vi "dfd_Render Real Root+.vi"(0 "Negative Exponent?":bool=TRUE, 4 "alignment(left, top)":T1, 5 "format string":string="%#g", 6 "bracket":cluster{"left":string, "right":string}={"left"="(", "right"=")"}, 7 "Fonts Input":T2(array[cluster]), 8 "variable":string="z", 9 "origin":cluster{"x":i16, "y":i16}, 10 "coefficients":dbl[](array[numeric]) format="%.2f", 11 "new picture":picture) -> (2 "text rect":T3, 3 "picture out":picture)   [LabVIEW 2017, in "NI_DigFilter_Process.lvlib"]
uses:
  <vilib>/addons/Digital Filter Design/NI_DigFilter_Process.lvlib
  <vilib>/Analysis/polynomials.llb/Unique Numbers and Multiplicity (DBL).vi
  <vilib>/Analysis/NI_AALPro.lvlib
panel:
  in  "Fonts Defaut":T2(array[cluster])=[{"Font Name:"="Tahoma", "Size"=13, "Strikeout?"=FALSE, "Italic?"=FALSE, "Underline?"=FALSE, "Outline?"=FALSE, "Shadow?"=FALSE, "Bold?"=FALSE}, {"Font Name:"="Tahoma", "Size"=13, "Strikeout?"=FALSE, "Italic?"=FALSE, "Underline?"=FALSE, "Outline?"=FALSE, "Shadow?"=FALSE, "Bold?"=FALSE}, {"Font Name:"="Tahoma", "Size"=11, "Strikeout?"=FALSE, "Italic?"=FALSE, "Underline?"=FALSE, "Outline?"=FALSE, "Shadow?"=FALSE, "Bold?"=FALSE}]
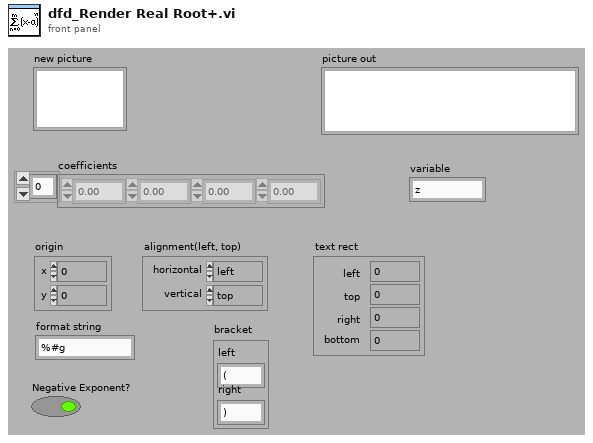
[diagram p1: front panel]
types:
  T1 = cluster{"horizontal":enum16{"left", "center", "right"}, "vertical":enum16{"top", "center", "bottom"}}
  T2 = cluster{"Font Name:":string, "Size":i16, "Strikeout?":bool, "Italic?":bool, "Underline?":bool, "Outline?":bool, "Shadow?":bool, "Bold?":bool}[]
  T3 = cluster{"left":i16, "top":i16, "right":i16, "bottom":i16}
  T4 = enum16{"User-specified Font", "Application Font", "System Font", "Dialog Font"}
  T5 = cluster{"Font Name:":string, "Size":i16, "Strikeout?":bool, "Italic?":bool, "Underline?":bool, "Outline?":bool, "Shadow?":bool, "Bold?":bool}
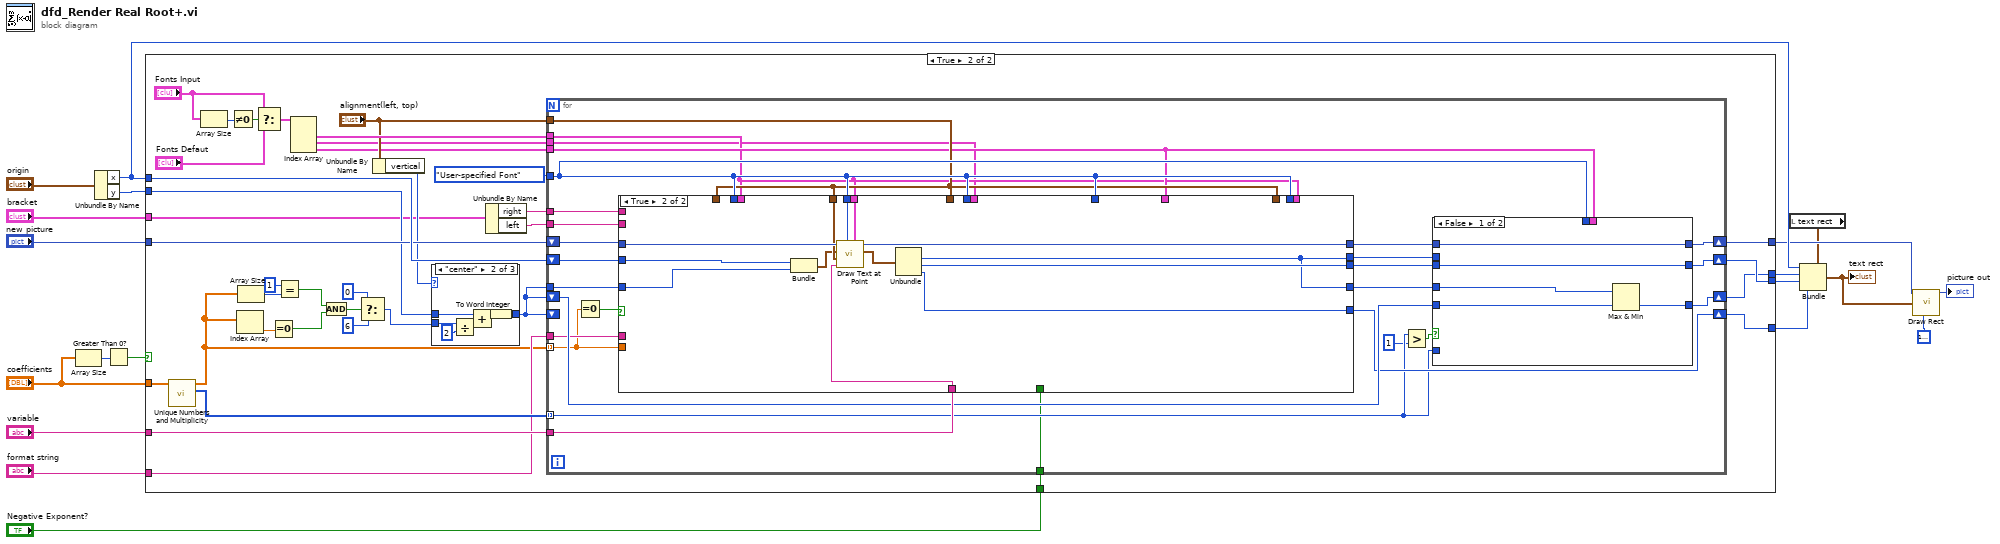
[diagram p0: block diagram]
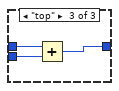
[diagram p4: hidden frame]
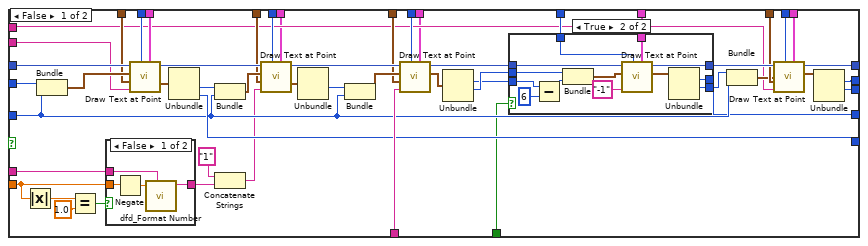
[diagram p5: hidden frame]
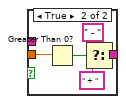
[diagram p7: hidden frame]
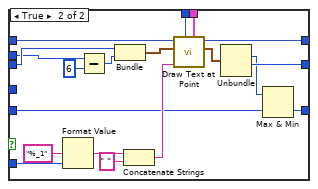
[diagram p8: hidden frame]
diagram:
  n1 = Array Size(array="coefficients") -> (size(s)=w12:i32)
  n2 = Unbundle By Name("origin") -> ("x"=w17:i16, "y"=w15:i16)
  n3 = Greater Than 0?(x=w12) -> (x > 0?=w11:bool)
  n4 = case shown="True" w11 {
    tunnel: [w22 w59] -> w19
    tunnel: [w21 w58] -> w18
    tunnel: w17 -> [w22 w56]
    tunnel: [w21 w55] -> w16
    tunnel: w15 -> [w21 w43]
    tunnel: [w20 w49] -> w7
    tunnel: "coefficients" -> [_ w47]
    tunnel: "new picture" -> [w20 w46]
    tunnel: "Negative Exponent?" -> [_ w38]
    tunnel: "variable" -> [_ w37]
    tunnel: "format string" -> [_ w36]
    tunnel: "bracket" -> [_ w35]
    frame False {
    }
    frame True {
      n5 = call-poly <vilib>:"Unique Numbers and Multiplicity.vi"("Numbers"=w47) -> ("Multiplicity"=w45:u32[], "Unique Numbers"=w32:dbl[])  [unwired: 9 out]
      n6 = Array Size(array="Fonts Input") -> (size(s)=w53:i32)
      n7 = Not Equal To 0?(x=w53) -> (x != 0?=w54:bool)
      n8 = Index Array(array=w32) -> (element=w31:dbl)  [unwired: 1 in]
      n9 = Array Size(array=w32) -> (size(s)=w30:i32)
      n10 = Select(t="Fonts Input", s=w54, f="Fonts Defaut") -> (s? t:f=w51:T2)
      n11 = Equal To 0?(x=w31) -> (x = 0?=w27:bool)
      n12 = Equal?(x=1, y=w30) -> (x = y?=w28:bool)
      n13 = Index Array(array=w51) -> (element #1=w48:T5, element #2=w40:T5, element #3=w39:T5)  [unwired: 3 in]
      n14 = And(x=w28, y=w27) -> (x .and. y?=w26:bool)
      n15 = Select(t=i16 0, s=w26, f=i16 6) -> (s? t:f=w24:i16)
      n16 = Unbundle By Name("alignment(left, top)") -> ("vertical"=w41:enum16{"top", "center", "bottom"})
      n17 = case shown="\"center\"" w41 {
        tunnel: [w60 w61 w68] -> w42
        tunnel: w43 -> [w60 w66 w69]
        tunnel: w24 -> [_ w64 w67]
        frame "bottom", Default {
        }
        frame "center" {
          n18 = Divide(x=w64, y=i16 2) -> (x/y=w62:dbl)
          n19 = Add(x=w66, y=w62) -> (x+y=w65:dbl)
          n20 = To Word Integer(number=w65) -> (16bit integer=w61:i16)
        }
        frame "top" {
          n21 = Add(x=w69, y=w67) -> (x+y=w68:i16)
        }
      }
      n22 = Unbundle By Name(w35) -> ("right"=w33:string, "left"=w34:string)
      n23 = for {
        tunnel: w32 -> [w81] mode=indexing
        shift-right: [w90] -> w49
        shift-left: w46 -> [w95]
        tunnel: w37 -> [w96]
        shift-right: [w89] -> w59
        shift-left: w56 -> [w94]
        tunnel: w42 -> [w92]
        shift-right: [w88] -> w58
        shift-left: w42 -> [w93]
        tunnel: T4."User-specified Font" ("desired font(Application)") -> [w80]
        shift-right: [w87] -> w55
        shift-left: w42 -> [_]
        tunnel: w36 -> [w91]
        tunnel: "alignment(left, top)" -> [w79]
        tunnel: w48 -> [w71]
        tunnel: w45 -> [w86] mode=indexing
        tunnel: w40 -> [w70]
        tunnel: w39 -> [w76]
        tunnel: w38 -> [w77]
        tunnel: w34 -> [w74]
        tunnel: w33 -> [w73]
        n24 = Equal To 0?(x=w81) -> (x = 0?=w78:bool)
        n25 = case shown="True" w78 {
          tunnel: w96 -> [w127 w185]
          tunnel: w79 -> [w128 _]
          tunnel: w95 -> [w147 w184]
          tunnel: w94 -> [w146 w180]
          tunnel: w92 -> [w111 w177]
          tunnel: w91 -> [w145 _]
          tunnel: [w123 w176] -> w87
          tunnel: [w117 w181] -> w85
          tunnel: [w115 w175] -> w84
          tunnel: w80 -> [w134 _]
          tunnel: w81 -> [w126 _]
          tunnel: w71 -> [w135 _]
          tunnel: w80 -> [w120 _]
          tunnel: w80 -> [w133 w182]
          tunnel: w80 -> [w132 _]
          tunnel: w79 -> [w131 _]
          tunnel: w79 -> [w129 w183]
          tunnel: w71 -> [w114 _]
          tunnel: w80 -> [w113 _]
          tunnel: w79 -> [w112 _]
          tunnel: w76 -> [w109 _]
          tunnel: w77 -> [w108 _]
          tunnel: [w106 w174] -> w75
          tunnel: w74 -> [w99 _]
          tunnel: w73 -> [w101 _]
          tunnel: [w100 w174] -> w72
          tunnel: w71 -> [w98 w173]
          tunnel: w70 -> [w97 _]
          frame False {
            n26 = Absolute Value(x=w126) -> (abs(x)=w107:dbl)
            n27 = Bundle("x"=w146, "y"=w111) -> (w138:cluster{"x":i16, "y":i16})  [unwired: 1 out]
            n28 = Equal?(x=w107, y=1.0) -> (x = y?=w124:bool)
            n29 = case shown="False" w124 {
              tunnel: w145 -> [w167 _]
              tunnel: [w166 w169] -> w104
              tunnel: w126 -> [w165 w170]
              frame False {
                n30 = Negate(x=w165) -> (-x=w164:dbl)
                n31 = call <vilib>:"dfd_Format Number.vi"("format string"=w167, "Coefficient"=w164) -> ("String Coefficient"=w166:string)  [unwired: 9 out]
              }
              frame True {
                n32 = Greater Than 0?(x=w170) -> (x > 0?=w171:bool)
                n33 = Select(t=" - " ("string"), s=w171, f=" + ") -> (s? t:f=w169:string)
              }
            }
            n34 = call <vilib>:"Draw Text at Point.vi"("[user-specified font]"=w135, "desired font(Application)"=w132, "text"=w99, "alignment(left, top)"=w131, "origin"=w138, "picture"=w147) -> ("text rect"=w142:T3, "new picture"=w143:picture)  [unwired: 3 in, 1 out]
            n35 = Unbundle(w142) -> ("right"=w140:i16, "bottom"=w123:i16)  [unwired: 2 out]
            n36 = Bundle("right"=w140, "y"=w111) -> (w130:cluster{"right":i16, "y":i16})  [unwired: 1 out]
            n37 = Concatenate Strings("1" ("string"), w104) -> (w102:string)
            n38 = call <vilib>:"Draw Text at Point.vi"("[user-specified font]"=w98, "desired font(Application)"=w133, "text"=w102, "alignment(left, top)"=w129, "origin"=w130, "picture"=w143) -> ("text rect"=w141:T3, "new picture"=w136:picture)  [unwired: 3 in, 1 out]
            n39 = Unbundle(w141) -> ("right"=w139:i16)  [unwired: 3 out]
            n40 = Bundle("right"=w139, "y"=w111) -> (w137:cluster{"right":i16, "y":i16})  [unwired: 1 out]
            n41 = call <vilib>:"Draw Text at Point.vi"("[user-specified font]"=w97, "desired font(Application)"=w134, "text"=w127, "alignment(left, top)"=w128, "origin"=w137, "picture"=w136) -> ("text rect"=w144:T3, "new picture"=w122:picture)  [unwired: 3 in, 1 out]
            n42 = Unbundle(w144) -> ("top"=w105:i16, "right"=w121:i16)  [unwired: 2 out]
            n43 = case shown="True" w108 {
              tunnel: w122 -> [w150 w159]
              tunnel: w121 -> [w149 w158]
              tunnel: w109 -> [_ w157]
              tunnel: [w150 w155] -> w118
              tunnel: [w149 w154] -> w116
              tunnel: w120 -> [_ w153]
              tunnel: [w148 w152] -> w106
              tunnel: w105 -> [w148 w151]
              frame False {
              }
              frame True {
                n44 = Subtract(x=w151, y=i16 6) -> (x-y=w162:i16)
                n45 = Bundle("right"=w158, w162) -> (w163:cluster{"right":i16, i16})  [unwired: 1 out]
                n46 = call <vilib>:"Draw Text at Point.vi"("[user-specified font]"=w157, "desired font(Application)"=w153, "text"="-1", "origin"=w163, "picture"=w159) -> ("text rect"=w160:T3, "new picture"=w155:picture)  [unwired: 4 in, 1 out]
                n47 = Unbundle(w160) -> ("top"=w152:i16, "right"=w154:i16)  [unwired: 2 out]
              }
            }
            n48 = Bundle("right"=w116, "y"=w111) -> (w110:cluster{"right":i16, "y":i16})  [unwired: 1 out]
            n49 = call <vilib>:"Draw Text at Point.vi"("[user-specified font]"=w114, "desired font(Application)"=w113, "text"=w101, "alignment(left, top)"=w112, "origin"=w110, "picture"=w118) -> ("text rect"=w119:T3, "new picture"=w117:picture)  [unwired: 3 in, 1 out]
            n50 = Unbundle(w119) -> ("top"=w100:i16, "right"=w115:i16)  [unwired: 2 out]
          }
          frame True {
            n51 = Bundle("x"=w180, "y"=w177) -> (w179:cluster{"x":i16, "y":i16})  [unwired: 1 out]
            n52 = call <vilib>:"Draw Text at Point.vi"("[user-specified font]"=w173, "desired font(Application)"=w182, "text"=w185, "alignment(left, top)"=w183, "origin"=w179, "picture"=w184) -> ("text rect"=w178:T3, "new picture"=w181:picture)  [unwired: 3 in, 1 out]
            n53 = Unbundle(w178) -> ("top"=w174:i16, "right"=w175:i16, "bottom"=w176:i16)  [unwired: 1 out]
          }
        }
        n54 = Greater?(x=w86, y=u32 1) -> (0:w82:bool)
        n55 = case shown="False" w82 {
          tunnel: w84 -> [w189 w208]
          tunnel: w76 -> [_ w207]
          tunnel: w85 -> [w190 w206]
          tunnel: w86 -> [_ w202]
          tunnel: [w190 w201] -> w90
          tunnel: [w189 w200] -> w89
          tunnel: w93 -> [w188 w195]
          tunnel: [w187 w193] -> w88
          tunnel: w80 -> [_ w192]
          tunnel: w75 -> [w186 _]
          tunnel: w72 -> [_ w191]
          frame False {
            n56 = Max & Min(x=w186, y=w188) -> (min(x,y)=w187:i16)  [unwired: 1 out]
          }
          frame True {
            n57 = Format Value(format string="%_1", value (0)=w202) -> (output string=w198:string)  [unwired: 1 out]
            n58 = Subtract(x=w191, y=i16 6) -> (x-y=w204:i16)
            n59 = Bundle("right"=w208, w204) -> (w203:cluster{"right":i16, i16})  [unwired: 1 out]
            n60 = Concatenate Strings(w198, " " ("string")) -> (w196:string)
            n61 = call <vilib>:"Draw Text at Point.vi"("[user-specified font]"=w207, "desired font(Application)"=w192, "text"=w196, "origin"=w203, "picture"=w206) -> ("text rect"=w209:T3, "new picture"=w201:picture)  [unwired: 4 in, 1 out]
            n62 = Unbundle(w209) -> ("top"=w194:i16, "right"=w200:i16)  [unwired: 2 out]
            n63 = Max & Min(x=w194, y=w195) -> (min(x,y)=w193:i16)  [unwired: 1 out]
          }
        }
      }
    }
  }
  n64 = local read "text rect"() -> (w1:T3)
  n65 = Bundle(cluster=w1, "left"=w17, "top"=w18, "right"=w19, "bottom"=w16) -> (w8:T3)
  "text rect" <- w8
  n66 = call <vilib>:"Draw Rect.vi"("picture"=w7, "rect"=w8, "color(black)"=u32 16777216) -> ("new picture"=→"picture out":picture)  [unwired: 2 in, 4 out]
